vi "Delete.vi"(8 "error in (no error)":errorcluster, 11 "Child Class in":refnum<class "Application.lvclass">) -> (0 "error out":errorcluster, 3 "Child Class out":refnum<class "Application.lvclass">)   [LabVIEW 2017, in "Application.lvlib" / "Application.lvclass"]
uses:
  Application.lvclass
  Application.lvclass/Application.ctl
  Settings/App Settings.lvclass
  Properties/App Properties.lvclass
  <vilib>/TSS/ACRObat Test Framework/Classes/Variable Engine/Class/Variable Engine.lvclass
  C:/Program Files (x86)/National Instruments/LabVIEW 2017/vi.lib/TSS/ACRObat Test Framework/Classes/Base Objects/Base Class/Base Class/Base Class.lvclass
  <vilib>/TSS/ACRObat Test Framework/Classes/Base Objects/Base Class/Base Class/Base Class.lvclass
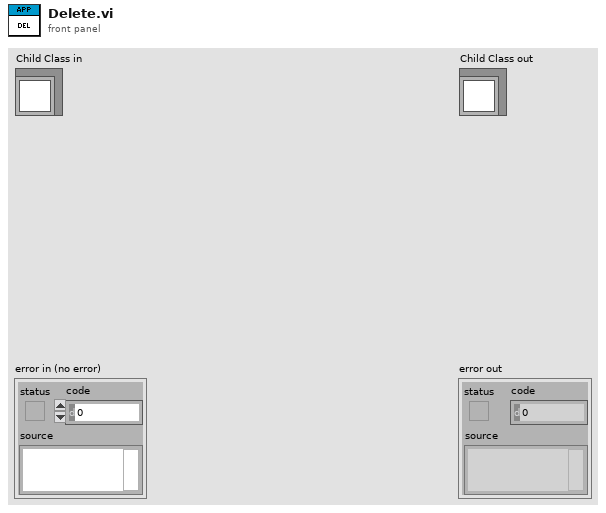
[diagram p1: front panel]
types:
  T1 = typedef "Application.lvlib/App Properties.lvclass/Class Properties -- Cluster.ctl" = cluster{"UUT Info":T2[], "Test Information":refnum<vi>, "Gold Board":refnum<class "Golden Board.lvclass">, "Test Recipe":refnum<class "Test Recipe.lvclass">, "Instruments":refnum<class "Instrument.lvclass">[], "Mode":T3, "Test Results":T4[], "Station Config":refnum<class "Station Config.lvclass">, "Variable Engine":refnum<class "Variable Engine.lvclass">}
  T2 = typedef "Application.lvlib/App Properties.lvclass/UUT Reference -- Cluster.ctl" = cluster{"Serial Number Reference":refnum<vi>, "Status Message Reference":refnum<vi>}
  T3 = typedef "Application.lvlib/Application.lvclass/Op Mode -- Enum.ctl" = u16
  T4 = typedef "Application.lvlib/App Properties.lvclass/Test Result -- Cluster.ctl" = cluster{"Position":i32, "Pass":bool, "Fail Codes":string}
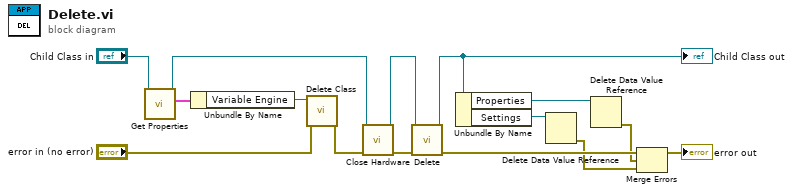
[diagram p0: block diagram]
diagram:
  n1 = call "Get Properties.vi"("Acrobat Template in"="Child Class in") -> ("Class Properties"=w4:T1, "Acrobat Template out"=w5:refnum<class "Application.lvclass">)  [unwired: 8 in, 1 out]
  n2 = Unbundle By Name(w4) -> ("Variable Engine"=w3:refnum<class "Variable Engine.lvclass">)
  n3 = call <vilib>:"Delete Class.vi"("error in (no error)"="error in (no error)", "Base Class in"=w3) -> ("error out"=w1:errorcluster)  [unwired: 8 in, 1 out]
  n4 = call-dynamic "Close Hardware.vi"("error in (no error)"=w1, "Application in"=w5) -> ("error out"=w10:errorcluster, "Application out"=w9:refnum<class "Application.lvclass">)  [unwired: 8 in]
  n5 = call-parent "Delete.vi"("error in (no error)"=w10, "Base Class in"=w9) -> ("error out"=w14:errorcluster, "Base Class out"=w15:refnum<class "Application.lvclass">)  [unwired: 8 in]
  "Child Class out" <- w15
  n6 = Unbundle By Name(w15) -> ("Properties"=w13:refnum<data-value>, "Settings"=w8:refnum<data-value>)
  n7 = Delete Data Value Reference(data value reference=w8) -> (error out=w7:errorcluster)  [unwired: 1 in, 1 out]
  n8 = Delete Data Value Reference(data value reference=w13) -> (error out=w11:errorcluster)  [unwired: 1 in, 1 out]
  n9 = Merge Errors(w14, w11, w7) -> (→"error out":errorcluster)
